vi "MotorControlWithBrake.vi"(6 "Brake Config":T1, 8 "Brake Engaged?":bool, 9 "Motor Cmd":dbl, 10 "BrakeDevRef":T2={"DeviceStatus"={"status"=FALSE, "code"=0, "source"=""}, "PWM Channel"=enum."Invalid", "DeadBand"={"Name"="", "maxPositivePwm"=0, "minPositivePwm"=0, "centerPwm"=0, "maxNegativePwm"=0, "minNegativePwm"=0, "angularRange"=0}}, 11 "MotorDevRef":T5={"DeviceStatus"={"status"=FALSE, "code"=0, "source"=""}, "Type"=enum."PWM", "PWM"={"PWM Channel"=enum."PWM 1", "DeadBand"={"Name"="", "maxPositivePwm"=0, "minPositivePwm"=0, "centerPwm"=0, "maxNegativePwm"=0, "minNegativePwm"=0, "angularRange"=0}}, "CAN"={"Device Number"=0, "SetOutput VI Ref"=variant(enum8{"Percent VBus", "Current", "Speed", "Position", "Voltage"} enum."Percent VBus"), "GetOutput VI Ref"=variant(refnum<k1> refnum), "Enable VI Ref"=variant(dbl 12.0), "Disable VI Ref"=variant(enum8{"Percent VBus", "Speed", "Position", "Slave", "Unchanged / Invalid", "Voltage Compensation", "Current", "Motion Profile"} enum."Percent VBus"), "Data"=variant}, "Invert"=FALSE, "DIO PWM"={"PWM \"Enable\" Channel"=enum."Invalid", "DIOChannel"=enum."Invalid", "PWM Rate"=0.0}}) -> ()   [LabVIEW 2017]
uses:
  BrakeMotorStates.ctl
  <vilib>/Rock Robotics/WPI/ThirdParty/Phoenix-LabVIEW/Motor Controller/Controls/CTRE_Phoenix_MotorControl_ControlMode.ctl
  <vilib>/Rock Robotics/SystemInterfaces/DIO/FPGA_DIOPWMChannel.ctl
  <vilib>/Rock Robotics/WPI/PWM/WPI_PWMDeadband.ctl
  <vilib>/Rock Robotics/WPI/MotorControl/WPI_MotorControlType.ctl
  <vilib>/Rock Robotics/SystemInterfaces/DIO/FPGA_DIOChannel.ctl
  <vilib>/Rock Robotics/WPI/MotorControl/WPI_MotorControlDeviceRef.ctl
  <vilib>/Rock Robotics/WPI/PWM/Servo/WPI_ServoDeviceRef.ctl
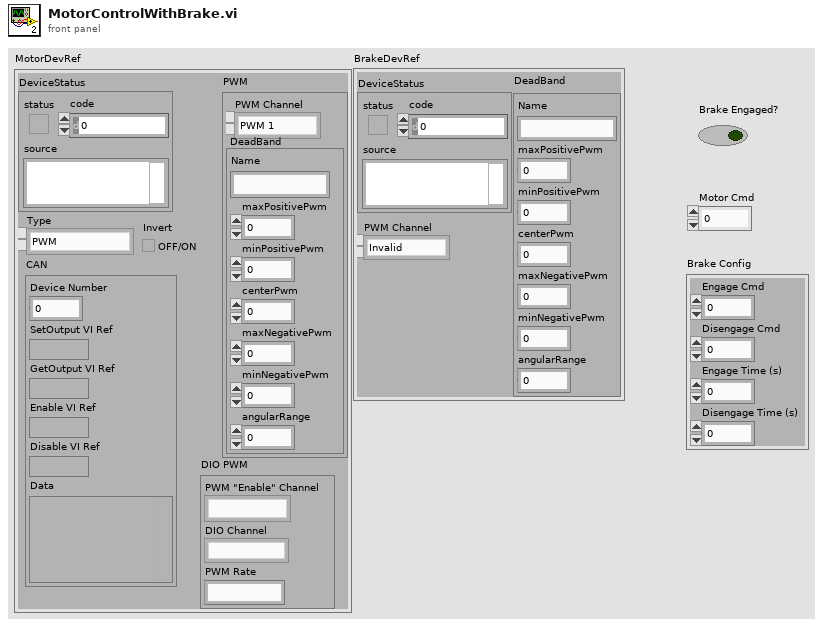
[diagram p1: front panel]
types:
  T1 = cluster{"Engage Cmd":dbl, "Disengage Cmd":dbl, "Engage Time (s)":dbl, "Disengage Time (s)":dbl}
  T2 = typedef "WPI_ServoDeviceRef.ctl" = cluster{"DeviceStatus":errorcluster, "PWM Channel":T3, "DeadBand":T4}
  T3 = typedef "FPGA_DIOPWMChannel.ctl" = enum8{"PWM 0", "PWM 1", "PWM 2", "PWM 3", "PWM 4", "PWM 5", "PWM 6", "PWM 7", "PWM 8", "PWM 9", "PWM MXP 0", "PWM MXP 1", "PWM MXP 2", "PWM MXP 3", "PWM MXP 4", "PWM MXP 5", "PWM MXP 6", "PWM MXP 7", "PWM MXP 8", "PWM MXP 9", "Invalid"}
  T4 = typedef "WPI_PWMDeadband.ctl" = cluster{"Name":string, "maxPositivePwm":i32, "minPositivePwm":i32, "centerPwm":i32, "maxNegativePwm":i32, "minNegativePwm":i32, "angularRange":u16}
  T5 = typedef "WPI_MotorControlDeviceRef.ctl" = cluster{"DeviceStatus":errorcluster, "Type":T6, "PWM":cluster{"PWM Channel":T3, "DeadBand":T4}, "CAN":cluster{"Device Number":u8, "SetOutput VI Ref":variant, "GetOutput VI Ref":variant, "Enable VI Ref":variant, "Disable VI Ref":variant, "Data":variant}, "Invert":bool, "DIO PWM":cluster{"PWM \"Enable\" Channel":T3, "DIOChannel":T7, "PWM Rate":dbl}}
  T6 = typedef "WPI_MotorControlType.ctl" = enum16{"PWM", "CAN", "DIO PWM"}
  T7 = typedef "FPGA_DIOChannel.ctl" = enum8{"DIO 0", "DIO 1", "DIO 2", "DIO 3", "DIO 4", "DIO 5", "DIO 6", "DIO 7", "DIO 8", "DIO 9", "DIO MXP 0", "DIO MXP 1", "DIO MXP 2", "DIO MXP 3", "DIO MXP 4", "DIO MXP 5", "DIO MXP 6", "DIO MXP 7", "DIO MXP 8", "DIO MXP 9", "DIO MXP 10", "DIO MXP 11", "DIO MXP 12", "DIO MXP 13", "DIO MXP 14", "DIO MXP 15", "SPI Port CS1", "SPI Port CS2", "SPI Port CS3", "SPI Port MISO", "SPI Port MOSI", "Invalid"}
  T8 = typedef "BrakeMotorStates.ctl" = enum16{"Engaged", "Disengaged", "Engage", "Disengage"}
  T9 = typedef "CTRE_Phoenix_MotorControl_ControlMode.ctl" = u16
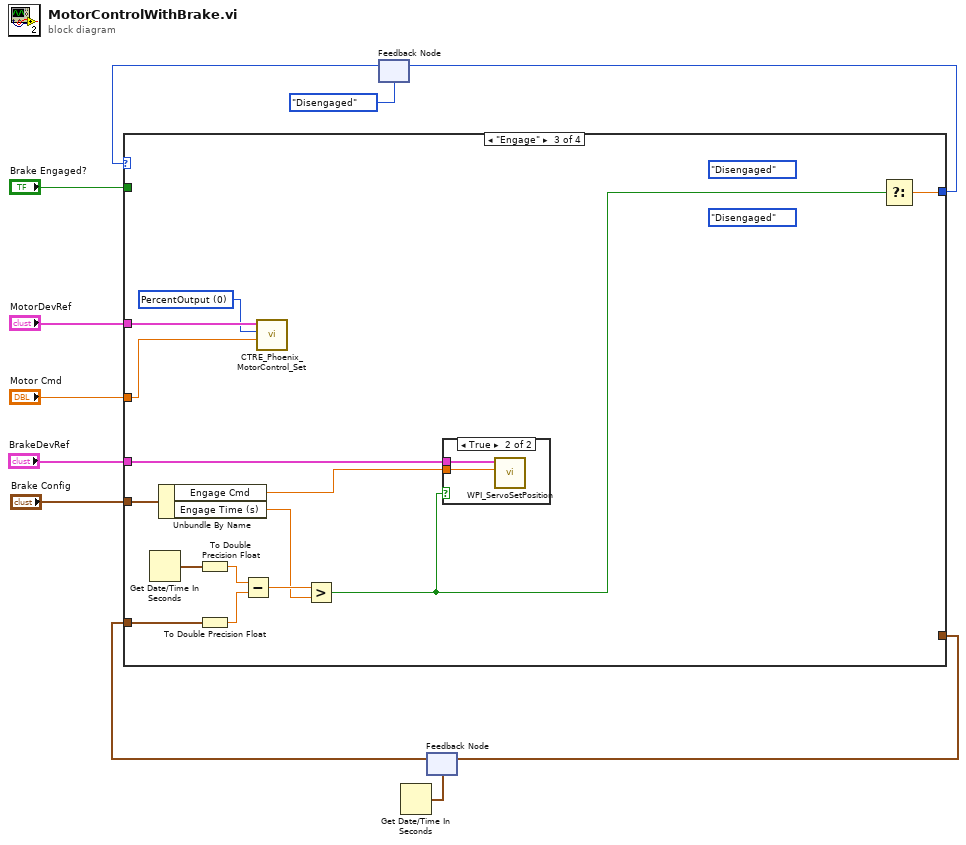
[diagram p0: block diagram]
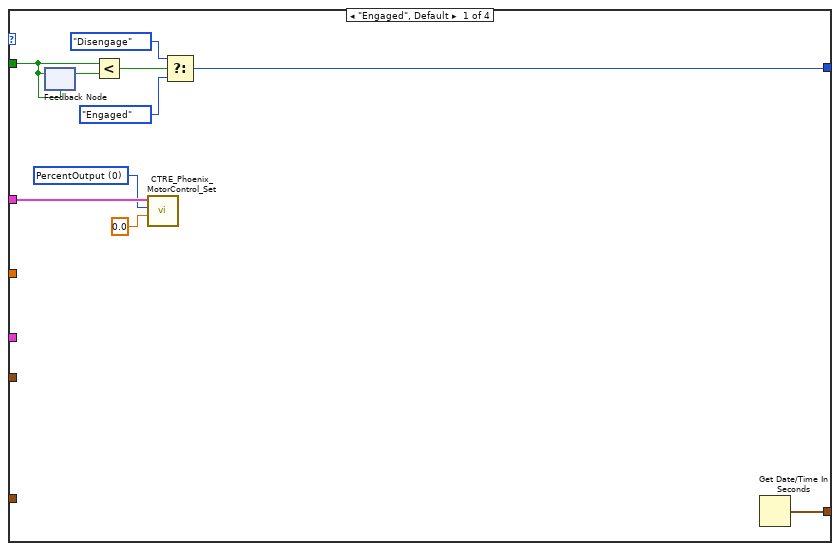
[diagram p2: hidden frame]
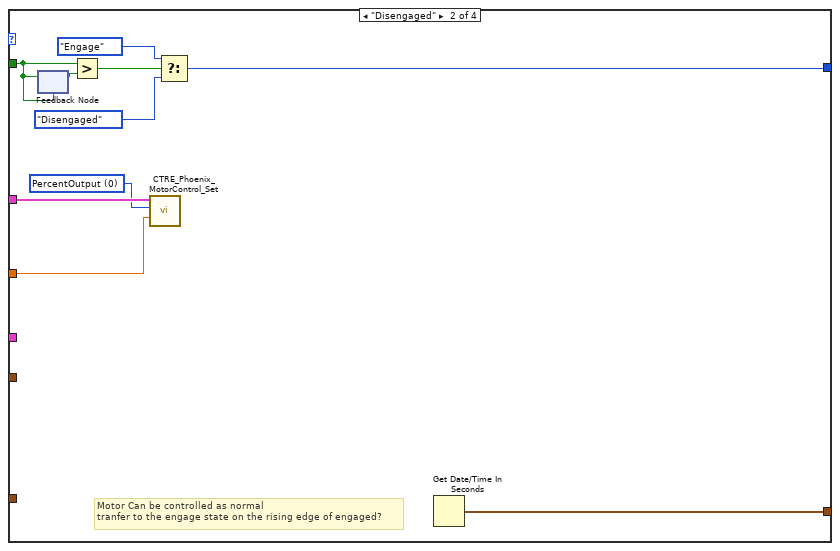
[diagram p3: hidden frame]
diagram:
  n1 = feedback #1(BrakeMotorStates."Disengaged") -> (w10:T8)
  n2 = Get Date/Time In Seconds() -> (seconds since 1Jan1904=w5:timestamp)
  n3 = feedback #2(w5) -> (w6:timestamp)
  n4 = case shown="\"Engage\"" w10 {
    tunnel: "MotorDevRef" -> [w21 w31 w45 _]
    tunnel: "Motor Cmd" -> [_ w29 w44 _]
    tunnel: [w18 w28 _ _] -> w7
    tunnel: w6 -> [_ _ w41 _]
    tunnel: "Brake Engaged?" -> [w16 w26 _ _]
    tunnel: [w12 w22 w33 _] -> w3
    tunnel: "Brake Config" -> [_ _ w37 _]
    tunnel: "BrakeDevRef" -> [_ _ w35 _]
    frame "Engaged", Default {
      w20 = T9 0 items=["PercentOutput"=0, "Position"=1, "Velocity"=2, "Current"=3, "Follower"=5, "MotionProfile"=6, "MotionMagic"=7, "MotionMagicArc"=8, "MotionProfileArc"=10, "Disabled"=15] ("Control Mode")
      n5 = feedback-in #3(w16) -> ()
      n6 = feedback #3(w16) -> (w17:bool)
      n7 = Less?(x=w16, y=w17) -> (x < y?=w15:bool)
      n8 = call <vilib>:"CTRE_Phoenix_MotorControl_Set.vi"("Output"=0.0, "Control Mode"=w20, "PhoenixMotorControlDevRef"=w21) -> ()  [unwired: 7 in, 2 out]
      n9 = Select(t=BrakeMotorStates."Disengage", s=w15, f=BrakeMotorStates."Engaged") -> (s? t:f=w12:T8)
      n10 = Get Date/Time In Seconds() -> (seconds since 1Jan1904=w18:timestamp)
    }
    frame "Disengaged" {
      w30 = T9 0 items=["PercentOutput"=0, "Position"=1, "Velocity"=2, "Current"=3, "Follower"=5, "MotionProfile"=6, "MotionMagic"=7, "MotionMagicArc"=8, "MotionProfileArc"=10, "Disabled"=15] ("Control Mode")
      # "Motor Can be controlled as normal\ntranfer to the engage state on the rising edge of engaged?"
      n11 = feedback-in #4(w26) -> ()
      n12 = feedback #4(w26) -> (w27:bool)
      n13 = Greater?(x=w26, y=w27) -> (0:w25:bool)
      n14 = call <vilib>:"CTRE_Phoenix_MotorControl_Set.vi"("Output"=w29, "Control Mode"=w30, "PhoenixMotorControlDevRef"=w31) -> ()  [unwired: 7 in, 2 out]
      n15 = Select(t=BrakeMotorStates."Engage", s=w25, f=BrakeMotorStates."Disengaged") -> (s? t:f=w22:T8)
      n16 = Get Date/Time In Seconds() -> (seconds since 1Jan1904=w28:timestamp)
    }
    frame "Engage" {
      (unwired) BrakeMotorStates."Disengaged"
      (unwired) BrakeMotorStates."Disengaged"
      w43 = T9 0 items=["PercentOutput"=0, "Position"=1, "Velocity"=2, "Current"=3, "Follower"=5, "MotionProfile"=6, "MotionMagic"=7, "MotionMagicArc"=8, "MotionProfileArc"=10, "Disabled"=15] ("Control Mode")
      n17 = Get Date/Time In Seconds() -> (seconds since 1Jan1904=w42:timestamp)
      n18 = Unbundle By Name(w37) -> ("Engage Cmd"=w34:dbl, "Engage Time (s)"=w36:dbl)
      n19 = To Double Precision Float(number=w42) -> (double precision float=w40:dbl)
      n20 = To Double Precision Float(number=w41) -> (double precision float=w39:dbl)
      n21 = Subtract(x=w40, y=w39) -> (x-y=w38:dbl)
      n22 = call <vilib>:"CTRE_Phoenix_MotorControl_Set.vi"("Output"=w44, "Control Mode"=w43, "PhoenixMotorControlDevRef"=w45) -> ()  [unwired: 7 in, 2 out]
      n23 = Greater?(x=w38, y=w36) -> (0:w32:bool)
      n24 = case shown="True" w32 {
        tunnel: w35 -> [_ w47]
        tunnel: w34 -> [_ w46]
        frame False {
        }
        frame True {
          n25 = call <vilib>:"WPI_ServoSetPosition.vi"("Position"=w46, "ServoDeviceRef"=w47) -> ()  [unwired: 8 in, 2 out]
        }
      }
      n26 = Select(s=w32) -> (s? t:f=w33:dbl)  [unwired: 2 in]
    }
    frame "Disengage" {
    }
  }
  n27 = feedback-in #1(w3) -> ()
  n28 = feedback-in #2(w7) -> ()
